vi "Build Command Line Arguments.vi"(10 "Arguments":string[](array[string]), 11 "Executable File Name":string="Revert to Scan Mode.exe") -> (3 "Command Line":string)   [LabVIEW 2019, in "SEECD System Explorer.lvlib"]
uses:
  SEECD System Explorer.lvlib
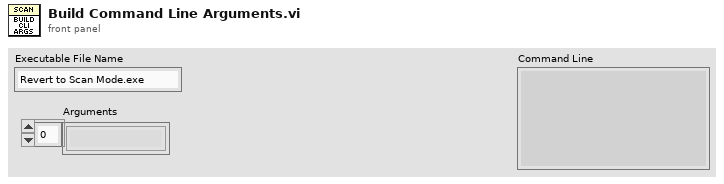
[diagram p1: front panel]
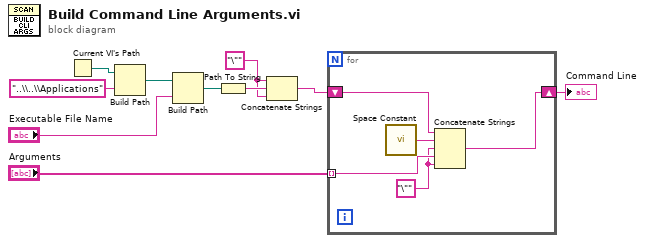
[diagram p0: block diagram]
diagram:
  w1 = "\""
  n1 = Current VI's Path() -> (path=w10:path)
  n2 = Build Path(base path=w10, name or relative path="..\\..\\Applications") -> (appended path=w5:path)
  n3 = Build Path(base path=w5, name or relative path="Executable File Name") -> (appended path=w6:path)
  n4 = Path To String(path=w6) -> (string=w8:string)
  n5 = Concatenate Strings(w1, w8, w1) -> (w3:string)
  n6 = for {
    tunnel: "Arguments" -> [w13] mode=indexing
    shift-right: [w14] -> w2
    shift-left: w3 -> [w15]
    w12 = "\""
    n7 = call <vilib>:"Space Constant.vi"() -> ("String"=w11:string)
    n8 = Concatenate Strings(w15, w11, w12, w13, w12) -> (w14:string)
  }
  "Command Line" <- w2
